vi "Write IntegrationTime.vi"(8 "error in (no error)":errorcluster, 10 "IntegrationTime":dbl=0.002, 11 "ElectrometerInternalConfiguration in":refnum<class "ElectrometerInternalConfiguration.lvclass">) -> (0 "error out":errorcluster, 3 "ElectrometerInternalConfiguration out":refnum<class "ElectrometerInternalConfiguration.lvclass">)   [LabVIEW 2016, in "ElectrometerInternalConfiguration.lvclass"]
uses:
  ElectrometerInternalConfiguration.lvclass
  ElectrometerInternalConfiguration.lvclass/ElectrometerInternalConfiguration.ctl
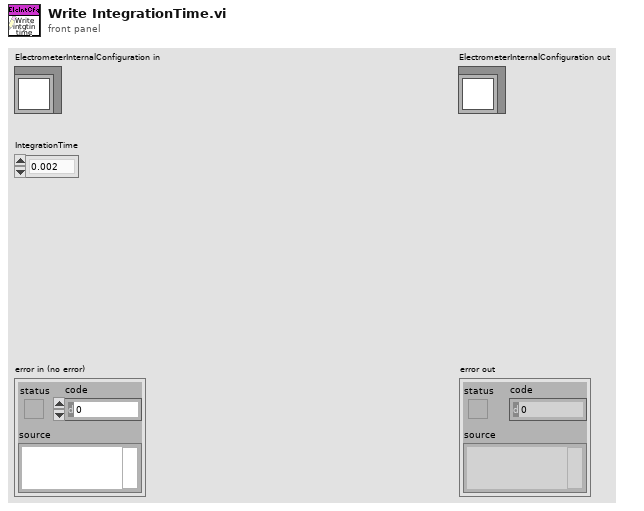
[diagram p1: front panel]
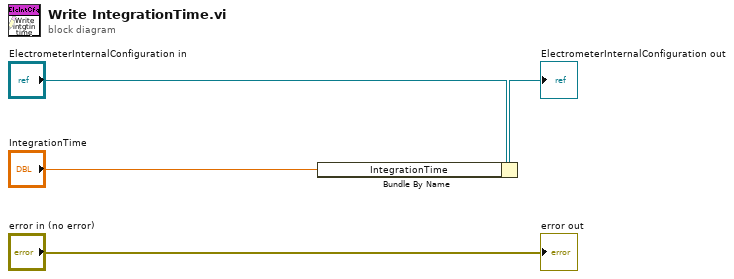
[diagram p0: block diagram]
diagram:
  n1 = Bundle By Name(cluster="ElectrometerInternalConfiguration in", "IntegrationTime"="IntegrationTime") -> (→"ElectrometerInternalConfiguration out":refnum<class "ElectrometerInternalConfiguration.lvclass">)
  "error out" <- "error in (no error)"
